vi "test-quintic-spline-06.vi"() -> (3 "Test Passed":bool)   [LabVIEW 2019]
uses:
  <vilib>/Rock Robotics/WPI/ThirdParty/JAS_Junk/TrajLib/POSEwCURVATURE.ctl
  <vilib>/Rock Robotics/WPI/ThirdParty/JAS_Junk/TrajLib/POSE2D.ctl
  <vilib>/Rock Robotics/WPI/ThirdParty/JAS_Junk/TrajLib/TRANSLATION2D.ctl
  <vilib>/Rock Robotics/WPI/ThirdParty/JAS_Junk/TrajLib/ROTATION2D.ctl
  <vilib>/Rock Robotics/WPI/ThirdParty/JAS_Junk/TrajLib/Rotation_CreateAngle.vi
  <vilib>/Rock Robotics/WPI/ThirdParty/JAS_Junk/TrajLib/Translation_Create.vi
  <vilib>/Rock Robotics/WPI/ThirdParty/JAS_Junk/TrajLib/Util_CalcDist.vi
  <vilib>/Rock Robotics/WPI/ThirdParty/JAS_Junk/TrajLib/Trajectory_Library.lvlib
panel:
  out "XY Graph":cluster{dbl[], dbl[]}(graph)
  out "Numb\nWaypoints":i32
  out "All Interior \nwayPoints\nFound (True)":bool
  out "end rot = 0":dbl
  out "end y = 0":dbl
  out "end x = 0":dbl
  out "start rot = 0":dbl
  out "start y = 0":dbl
  out "start x = 0":dbl
  out "max dtheta < 0.0872":dbl
  out "max dy < 0.00127":dbl
  out "max dx  < 0.127":dbl
  out "Overall Error":errorcluster
  out "Elements":i32
  out "Create Spline Error":errorcluster
  out "SplinePoses\nWCurve":T1[](array[typedef]) {"POSE"."ROTATION"."SIN" format="%13.4f"; "POSE"."ROTATION"."COS" format="%13.4f"; "POSE"."ROTATION"."VALUE" format="%13.4f"; "POSE"."TRANSLATION"."Y" format="%14.3f"; "POSE"."TRANSLATION"."X" format="%14.3f"}
  out "Elapsed Time":dbl
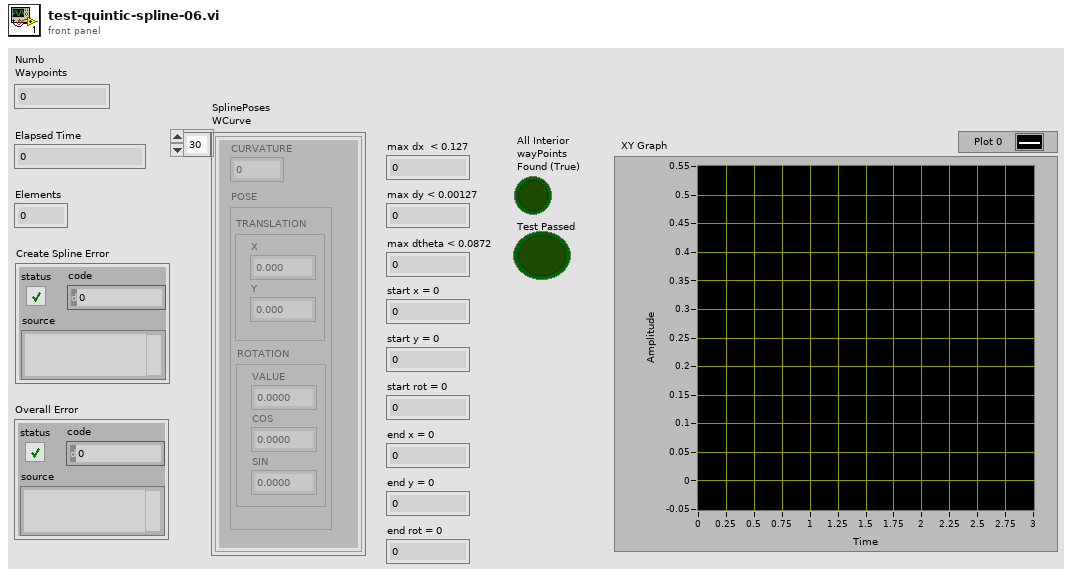
[diagram p1: front panel]
types:
  T1 = typedef "Trajectory_Library.lvlib/POSEwCURVATURE.ctl" = cluster{"CURVATURE":dbl, "POSE":T2}
  T2 = typedef "Trajectory_Library.lvlib/POSE2D.ctl" = cluster{"TRANSLATION":T3, "ROTATION":T4}
  T3 = typedef "Trajectory_Library.lvlib/TRANSLATION2D.ctl" = cluster{"X":dbl, "Y":dbl}
  T4 = typedef "Trajectory_Library.lvlib/ROTATION2D.ctl" = cluster{"VALUE":dbl, "COS":dbl, "SIN":dbl}
  T5 = typedef "Trajectory_Library.lvlib/SPLINE.ctl" = cluster{"Degree":i32, "Coefficients":T6}
  T6 = typedef "NI_Matrix.lvlib/RealMatrix.ctl" = dbl[][]
  T7 = typedef "Trajectory_Library.lvlib/TWIST2D.ctl" = cluster{"dX":dbl, "dY":dbl, "dTHETA":dbl}
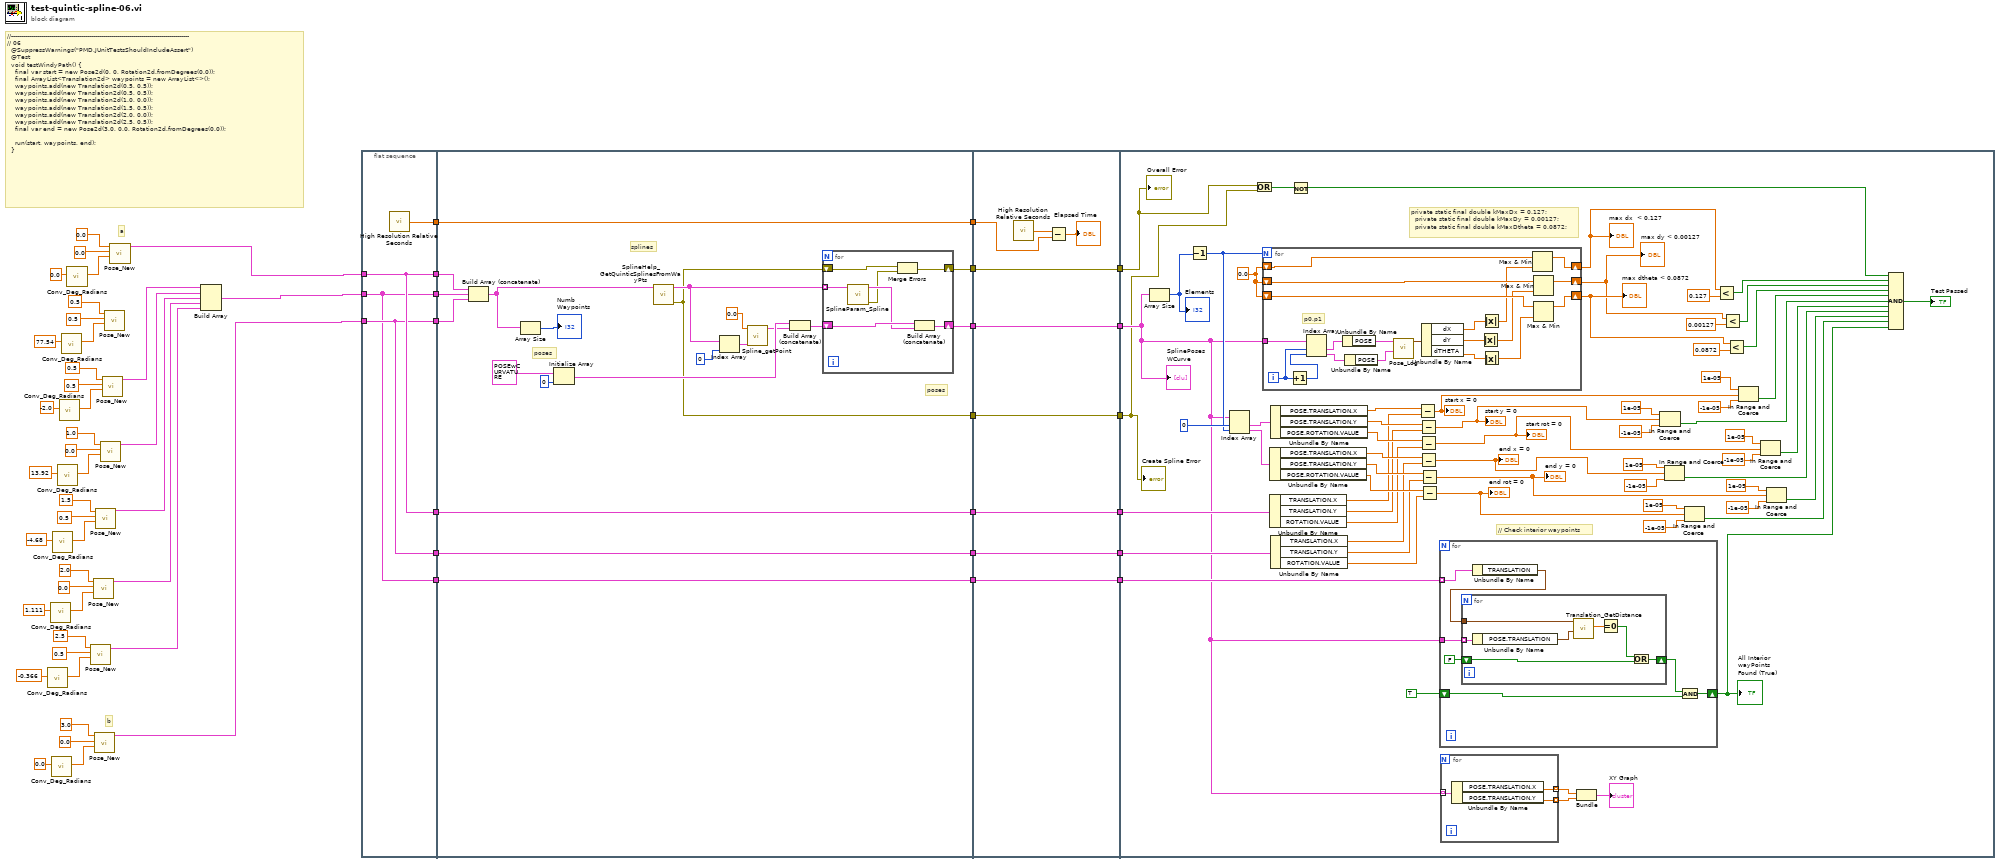
[diagram p0: block diagram]
diagram:
  # "b"
  # "a"
  # "//-----------------------------------------------------------------------------------------\n// 06\n  @SuppressWarnings(\"PMD.JUnitTestsShouldIncludeAssert\")\n  @Test\n  void testWindyPath() {\n    final var start = new Pose2d(0, 0, Rotation2d.fromDegrees(0.0));\n    final ArrayList<Translation2d> waypoints = new ArrayList<>();\n    waypoints.add(new Translation2d(0.5, 0.5));\n    waypoints.add(new Translation2d(0.5, 0.5));\n    waypoints.add(new Translation2d(1.0, 0.0));\n    waypoints.add(new Translation2d(1.5, 0.5));\n    waypoints.add(new Translation2d(2.0, 0.0));\n    waypoints.add(new Translation2d(2.5, 0.5));\n    final var end = new Pose2d(3.0, 0.0, Rotation2d.fromDegrees(0.0));\n\n    run(start, waypoints, end);\n  }"
  n1 = call <vilib>:"Conv_Deg_Radians.vi"("Degress"=-0.366) -> ("Radians"=w10:dbl)  [unwired: 10 in]
  n2 = call <vilib>:"Conv_Deg_Radians.vi"("Degress"=1.111) -> ("Radians"=w14:dbl)  [unwired: 10 in]
  n3 = call <vilib>:"Conv_Deg_Radians.vi"("Degress"=0.0) -> ("Radians"=w38:dbl)  [unwired: 10 in]
  n4 = call <vilib>:"Conv_Deg_Radians.vi"("Degress"=-4.68) -> ("Radians"=w18:dbl)  [unwired: 10 in]
  n5 = call <vilib>:"Conv_Deg_Radians.vi"("Degress"=13.92) -> ("Radians"=w22:dbl)  [unwired: 10 in]
  n6 = call <vilib>:"Conv_Deg_Radians.vi"("Degress"=-2.0) -> ("Radians"=w26:dbl)  [unwired: 10 in]
  n7 = call <vilib>:"Conv_Deg_Radians.vi"("Degress"=77.54) -> ("Radians"=w30:dbl)  [unwired: 10 in]
  n8 = call <vilib>:"Conv_Deg_Radians.vi"("Degress"=0.0) -> ("Radians"=w35:dbl)  [unwired: 10 in]
  n9 = call <vilib>:"Pose_New.vi"("Heading"=w10, "Y"=0.5, "X"=2.5) -> ("out POSe"=w4:T2)  [unwired: 8 in]
  n10 = call <vilib>:"Pose_New.vi"("Heading"=w14, "Y"=0.0, "X"=2.0) -> ("out POSe"=w5:T2)  [unwired: 8 in]
  n11 = call <vilib>:"Pose_New.vi"("Heading"=w38, "Y"=0.0, "X"=3.0) -> ("out POSe"=w1:T2)  [unwired: 8 in]
  n12 = call <vilib>:"Pose_New.vi"("Heading"=w18, "Y"=0.5, "X"=1.5) -> ("out POSe"=w6:T2)  [unwired: 8 in]
  n13 = call <vilib>:"Pose_New.vi"("Heading"=w22, "Y"=0.0, "X"=1.0) -> ("out POSe"=w7:T2)  [unwired: 8 in]
  n14 = call <vilib>:"Pose_New.vi"("Heading"=w26, "Y"=0.5, "X"=0.5) -> ("out POSe"=w8:T2)  [unwired: 8 in]
  n15 = call <vilib>:"Pose_New.vi"("Heading"=w30, "Y"=0.5, "X"=0.5) -> ()  [unwired: 8 in, 1 out]
  n16 = call <vilib>:"Pose_New.vi"("Heading"=w35, "Y"=0.0, "X"=0.0) -> ("out POSe"=w3:T2)  [unwired: 8 in]
  n17 = Build Array(w8, w7, w6, w5, w4) -> (w2:T2[])
  n18 = flat-sequence {
    tunnel: w3 -> [w63]
    tunnel: [w63] -> w60
    tunnel: w1 -> [w62]
    tunnel: [w62] -> w59
    tunnel: [w64] -> w58
    tunnel: [w63] -> w50
    tunnel: [w62] -> w47
    tunnel: [w61] -> w42
    tunnel: w2 -> [w61]
    tunnel: [w61] -> w41
    tunnel: w60 -> [w69]
    tunnel: w59 -> [w68]
    tunnel: [w85] -> w57
    tunnel: w58 -> [w85]
    tunnel: [w75] -> w56
    tunnel: [w74] -> w54
    tunnel: [w73] -> w52
    tunnel: w50 -> [w72]
    tunnel: [w72] -> w49
    tunnel: w47 -> [w71]
    tunnel: [w71] -> w46
    tunnel: [w70] -> w43
    tunnel: w42 -> [w70]
    tunnel: w41 -> [w66]
    tunnel: w57 -> [w101]
    tunnel: w56 -> [w100]
    tunnel: [w100] -> w55
    tunnel: w54 -> [w99]
    tunnel: [w99] -> w53
    tunnel: w52 -> [w98]
    tunnel: [w98] -> w51
    tunnel: w49 -> [w95]
    tunnel: [w95] -> w48
    tunnel: w46 -> [w94]
    tunnel: [w94] -> w45
    tunnel: [w93] -> w44
    tunnel: w43 -> [w93]
    tunnel: w55 -> [w142]
    tunnel: w53 -> [w130]
    tunnel: w51 -> [w129]
    tunnel: w48 -> [w164]
    tunnel: w45 -> [w163]
    tunnel: w44 -> [w146]
    frame #0 {
      n19 = call <vilib>:"High Resolution Relative Seconds.vi"() -> ("relative seconds"=w64:dbl)
    }
    frame #1 {
      # "poses"
      # "poses"
      # "splines"
      n20 = Build Array (concatenate)(w69, w66, w68) -> (w65:T2[])
      n21 = Array Size(array=w65) -> (size(s)=→"Numb\nWaypoints":i32)
      n22 = Initialize Array(T1 {"CURVATURE"=0.0, "POSE"={"TRANSLATION"={"X"=0.0, "Y"=0.0}, "ROTATION"={"VALUE"=0.0, "COS"=1.0, "SIN"=0.0}}} ("POSEwCURVATURE"), 0 ("dimension size")) -> (w79:T1[])
      n23 = call <vilib>:"SplineHelp_GetQuinticSplinesFromWayPts.vi"("WayPoints"=w65) -> ("out Error"=w74:errorcluster, "Splines"=w76:T5[])  [unwired: 9 in]
      n24 = Index Array(array=w76, index=0) -> (element=w81:T5)
      n25 = call <vilib>:"Spline_getPoint.vi"("inputSPLINE"=w81, "Time"=0.0) -> ("POSEwCURVATURE"=w78:T1)  [unwired: 9 in]
      n26 = Build Array (concatenate)(w79, w78) -> (w77:T1[])
      n27 = for {
        shift-right: [w89] -> w75
        shift-left: w77 -> [w91]
        tunnel: w76 -> [w92] mode=indexing
        shift-right: [w87] -> w73
        shift-left: w74 -> [w88]
        n28 = call <vilib>:"SplineParam_Spline.vi"("inputSPLINE"=w92) -> ("error out"=w86:errorcluster, "outputPOSEwCURVATURE"=w90:T1[])  [unwired: 9 in]
        n29 = Merge Errors(w88, w86) -> (w87:errorcluster)
        n30 = Build Array (concatenate)(w91, w90) -> (w89:T1[])
      }
    }
    frame #2 {
      n31 = call <vilib>:"High Resolution Relative Seconds.vi"() -> ("relative seconds"=w96:dbl)
      n32 = Subtract(x=w96, y=w101) -> (x-y=→"Elapsed Time":dbl)
    }
    frame #3 {
      w165 = 0.0
      # "// Check interior waypoints"
      # "private static final double kMaxDx = 0.127;\n  private static final double kMaxDy = 0.00127;\n  private static final double kMaxDtheta = 0.0872;"
      n33 = Array Size(array=w142) -> (size(s)=w166:i32)
      "Elements" <- w166
      n34 = Decrement(x=w166) -> (x-1=w161:i32)
      n35 = Index Array(array=w142, index #1=0 ("index"), index #2=w161) -> (element #1=w160:T1, element #2=w159:T1)
      n36 = Or(x=w129, y=w130) -> (x .or. y?=w131:bool)
      n37 = for {
        N: w161 -> [_]
        tunnel: w142 -> [w201]
        shift-right: [w192] -> w135
        shift-left: w165 -> [w189]
        shift-right: [w190] -> w137
        shift-left: w165 -> [w187]
        shift-right: [w191] -> w136
        shift-left: w165 -> [w188]
        i -> [w203]
        # "p0,p1"
        n38 = Increment(x=w203) -> (x+1=w202:i32)
        n39 = Index Array(array=w201, index #1=w203, index #2=w202) -> (element #1=w200:T1, element #2=w199:T1)
        n40 = Unbundle By Name(w200) -> ("POSE"=w198:T2)
        n41 = Unbundle By Name(w199) -> ("POSE"=w197:T2)
        n42 = call <vilib>:"Pose_Log.vi"("end POSE"=w197, "in POSE"=w198) -> ("out TWIST"=w196:T7)  [unwired: 9 in]
        n43 = Unbundle By Name(w196) -> ("dX"=w193:dbl, "dY"=w194:dbl, "dTHETA"=w195:dbl)
        n44 = Absolute Value(x=w194) -> (abs(x)=w185:dbl)
        n45 = Absolute Value(x=w193) -> (abs(x)=w186:dbl)
        n46 = Absolute Value(x=w195) -> (abs(x)=w184:dbl)
        n47 = Max & Min(x=w189, y=w186) -> (max(x,y)=w192:dbl)  [unwired: 1 out]
        n48 = Max & Min(x=w188, y=w185) -> (max(x,y)=w191:dbl)  [unwired: 1 out]
        n49 = Max & Min(x=w187, y=w184) -> (max(x,y)=w190:dbl)  [unwired: 1 out]
      }
      "max dx  < 0.127" <- w135
      "max dy < 0.00127" <- w136
      "max dtheta < 0.0872" <- w137
      n50 = Unbundle By Name(w159) -> ("POSE.TRANSLATION.X"=w155:dbl, "POSE.TRANSLATION.Y"=w154:dbl, "POSE.ROTATION.VALUE"=w153:dbl)
      n51 = Unbundle By Name(w164) -> ("TRANSLATION.X"=w152:dbl, "TRANSLATION.Y"=w151:dbl, "ROTATION.VALUE"=w150:dbl)
      n52 = Unbundle By Name(w160) -> ("POSE.TRANSLATION.X"=w158:dbl, "POSE.TRANSLATION.Y"=w157:dbl, "POSE.ROTATION.VALUE"=w156:dbl)
      n53 = Unbundle By Name(w163) -> ("TRANSLATION.X"=w149:dbl, "TRANSLATION.Y"=w148:dbl, "ROTATION.VALUE"=w147:dbl)
      n54 = Not(x=w131) -> (.not. x?=w128:bool)
      n55 = Subtract(x=w158, y=w152) -> (x-y=w124:dbl)
      "start x = 0" <- w124
      n56 = Subtract(x=w157, y=w151) -> (x-y=w103:dbl)
      "start y = 0" <- w103
      n57 = Subtract(x=w156, y=w150) -> (x-y=w107:dbl)
      "start rot = 0" <- w107
      n58 = Subtract(x=w155, y=w149) -> (x-y=w108:dbl)
      "end x = 0" <- w108
      n59 = Subtract(x=w154, y=w148) -> (x-y=w115:dbl)
      "end y = 0" <- w115
      n60 = Subtract(x=w153, y=w147) -> (x-y=w119:dbl)
      "end rot = 0" <- w119
      n61 = for {
        tunnel: w146 -> [w171] mode=indexing
        tunnel: w142 -> [w176]
        shift-right: [w175] -> w127
        shift-left: TRUE -> [w174]
        n62 = Unbundle By Name(w171) -> ("TRANSLATION"=w170:T3)
        n63 = for {
          tunnel: w176 -> [w180] mode=indexing
          shift-right: [w183] -> w172
          shift-left: FALSE -> [w182]
          tunnel: w170 -> [w181]
          n64 = Unbundle By Name(w180) -> ("POSE.TRANSLATION"=w179:T3)
          n65 = call <vilib>:"Translation_GetDistance.vi"("other Translation"=w179, "In Translation"=w181) -> ("Distance"=w178:dbl)  [unwired: 9 in]
          n66 = Equal To 0?(x=w178) -> (x = 0?=w177:bool)
          n67 = Or(x=w177, y=w182) -> (x .or. y?=w183:bool)
        }
        n68 = And(x=w172, y=w174) -> (x .and. y?=w175:bool)
      }
      "All Interior \nwayPoints\nFound (True)" <- w127
      n69 = for {
        tunnel: [w169] -> w144 mode=indexing
        tunnel: [w168] -> w143 mode=indexing
        tunnel: w142 -> [w167] mode=indexing
        n70 = Unbundle By Name(w167) -> ("POSE.TRANSLATION.X"=w169:dbl, "POSE.TRANSLATION.Y"=w168:dbl)
      }
      n71 = Bundle(w144, w143) -> (→"XY Graph":cluster{dbl[], dbl[]})  [unwired: 1 in]
      n72 = In Range and Coerce(upper limit=1e-05, x=w103, lower limit=-1e-05) -> (In Range?=w104:bool)  [unwired: 1 out]
      n73 = In Range and Coerce(upper limit=1e-05, x=w108, lower limit=-1e-05) -> (In Range?=w110:bool)  [unwired: 1 out]
      n74 = In Range and Coerce(upper limit=1e-05, x=w119, lower limit=-1e-05) -> (In Range?=w120:bool)  [unwired: 1 out]
      n75 = Less?(x=w135, y=0.127) -> (x < y?=w134:bool)
      n76 = Less?(x=w136, y=0.00127) -> (x < y?=w133:bool)
      n77 = Less?(x=w137, y=0.0872) -> (x < y?=w132:bool)
      n78 = In Range and Coerce(upper limit=1e-05, x=w124, lower limit=-1e-05) -> (In Range?=w123:bool)  [unwired: 1 out]
      n79 = In Range and Coerce(upper limit=1e-05, x=w107, lower limit=-1e-05) -> (In Range?=w109:bool)  [unwired: 1 out]
      n80 = In Range and Coerce(upper limit=1e-05, x=w115, lower limit=-1e-05) -> (In Range?=w116:bool)  [unwired: 1 out]
      n81 = Compound Arithmetic op=AND(w128, w134, w133, w132, w123, w104, w109, w110, w116, w120, w127) -> (→"Test Passed":bool)
      "SplinePoses\nWCurve" <- w142
      "Create Spline Error" <- w130
      "Overall Error" <- w129
    }
  }
